vi "Untitled 4.vi"() -> ()   [LabVIEW 2018]
uses:
  <vilib>/Utility/miscctls.llb/LVPointTypeDef.ctl
panel:
  in  "Origin":T1
  in  "Slide":dbl(slide) scale=0.0..1.0
  in  "stop":bool
  out "2D Picture":picture
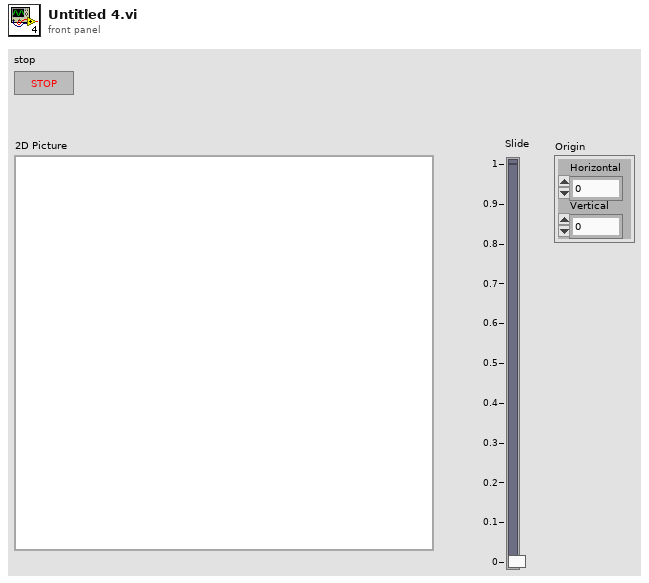
[diagram p1: front panel]
types:
  T1 = typedef "LVPointTypeDef.ctl" = cluster{"Horizontal":i16, "Vertical":i16}
  T2 = typedef "imagedata.ctl" = cluster{"image type":i32, "image depth":i32, "image":u8[], "mask":u8[], "colors":u32[], "Rectangle":cluster{"left":i16, "top":i16, "right":i16, "bottom":i16}}
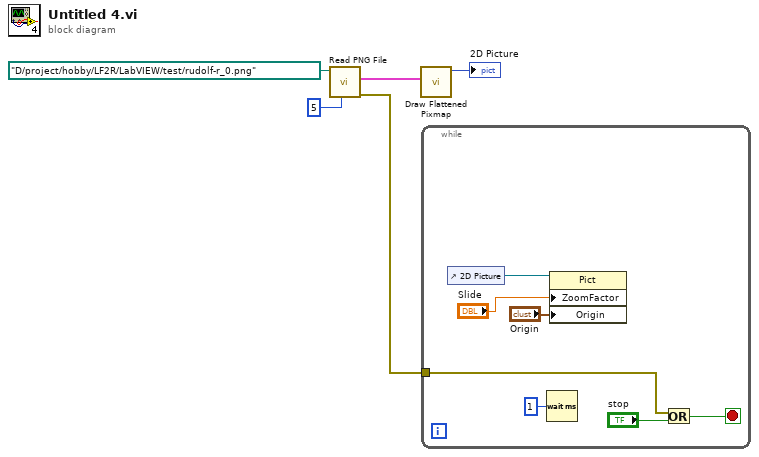
[diagram p0: block diagram]
diagram:
  n1 = call <vilib>:"Read PNG File.vi"("Transparency Thresh"=u8 5, "path to PNG file"=path "D:/project/hobby/LF2R/LabVIEW/test/rudolf-r_0.png") -> ("error out"=w1:errorcluster, "image data"=w4:T2)  [unwired: 7 in, 1 out]
  n2 = call <vilib>:"Draw Flattened Pixmap.vi"("image data"=w4) -> ("new picture"=→"2D Picture":picture)  [unwired: 8 in]
  n3 = while {
    tunnel: w1 -> [w11]
    stop <- w10 stop-if-true
    n4 = control-ref of="2D Picture"() -> (w8:refnum<vi>)
    n5 = Wait (ms)(milliseconds to wait=u32 1) -> ()  [unwired: 1 out]
    n6 = property class="Pict"(reference=w8, "ZoomFactor"="Slide", "Origin"="Origin") -> ()  [unwired: 1 in, 2 out]
    n7 = Or(x=w11, y="stop") -> (x .or. y?=w10:bool)
  }
